vi "Authority Management.vi"() -> ()   [LabVIEW 2017]
uses:
  <vilib>/Utility/error.llb/DialogType.ctl
  Controls/Login Authority CSV FGV Command.ctl
  <vilib>/Utility/file.llb/Read From Spreadsheet File (string).vi
  Globle/Trigger Home Screen.vi
panel:
  in  "Cancel Button - Archive":bool
  in  "Delete":bool
  out "error out":errorcluster
  in  "error in (no error)":errorcluster
  in  "New":bool
  in  "Save":bool
  in  "Enable Disable":T1
  in  "SELECT AUTHORITY":string(combo)
  # "AUTHORITY ASSIGNMENT"
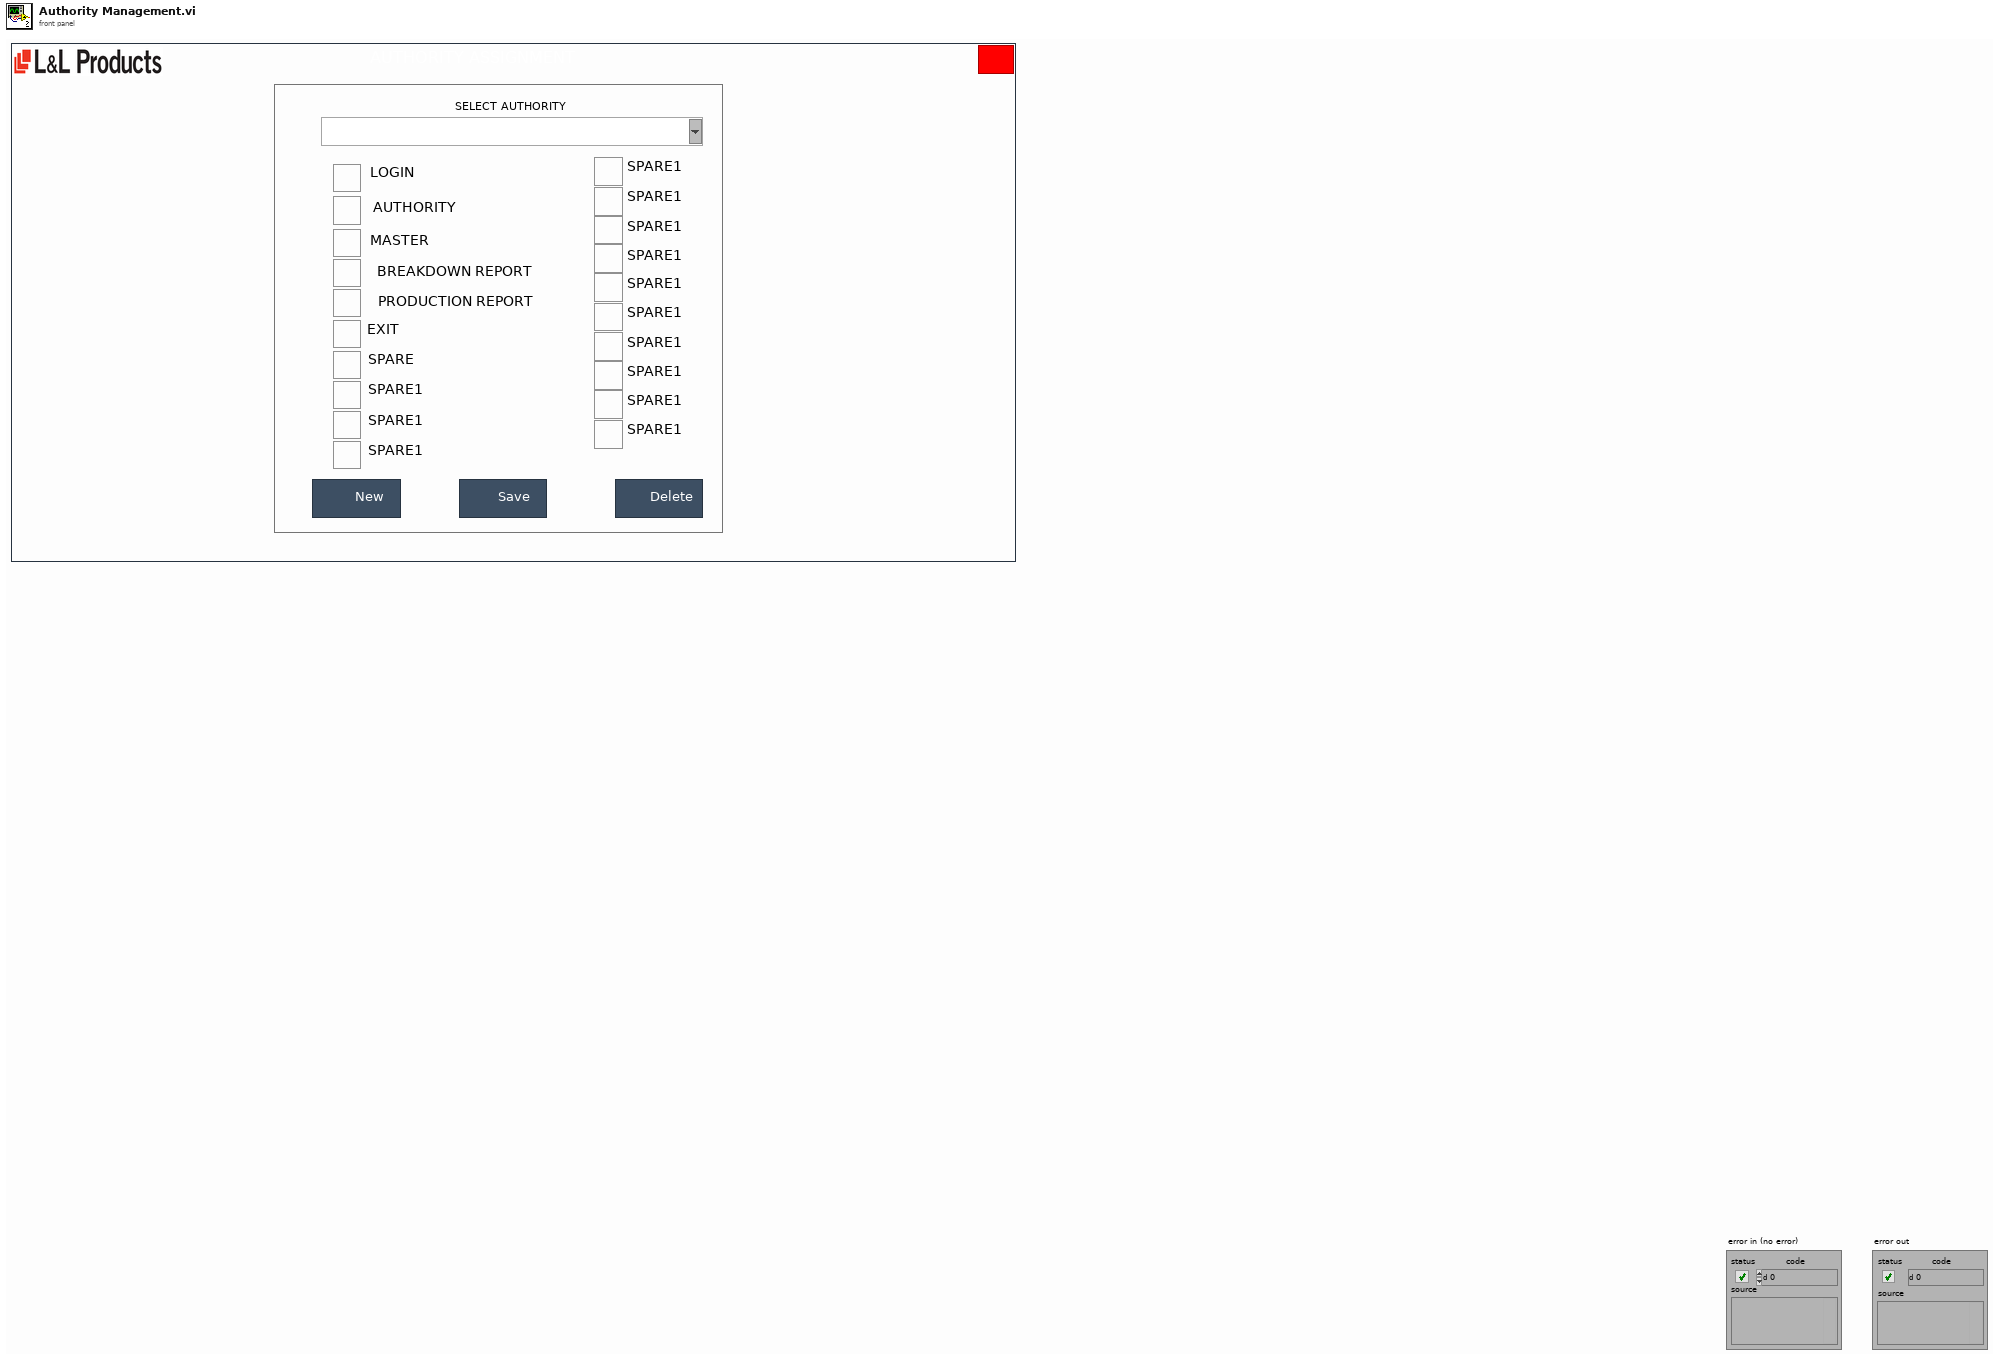
[diagram p1: front panel]
types:
  T1 = cluster{"SCREEN 1":bool, "SCREEN 2":bool, "SCREEN 3":bool, "SCREEN 4":bool, "SCREEN 5":bool, "SCREEN 6":bool, "SCREEN 7":bool, "SCREEN 8":bool, "SCREEN 9":bool, "SCREEN 10":bool, "SCREEN 11":bool, "SCREEN 12":bool, "SCREEN 13":bool, "SCREEN 14":bool, "SCREEN 15":bool, "SCREEN 16":bool, "SCREEN 17":bool, "SCREEN 18":bool, "SCREEN 19":bool, "SCREEN 20":bool}
  T2 = typedef "Login Authority CSV FGV Command.ctl" = enum16{"Init", "Save", "Read", "Get Data", "Delete"}
  T3 = typedef "DialogType.ctl" = u16
  T4 = enum32{"invalid app kind", "Development System", "Run Time System", "Student Edition", "Embedded LabVIEW", "Evaluation", "Custom"}
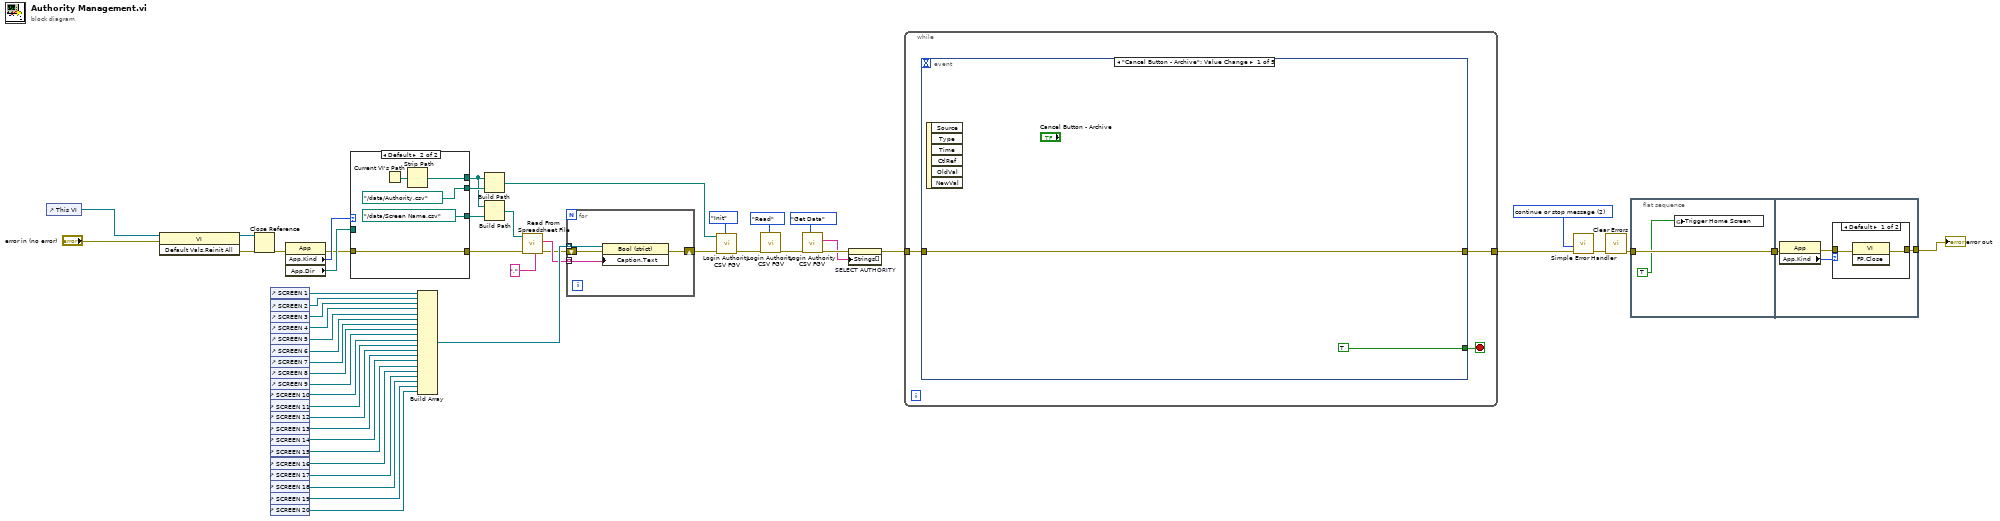
[diagram p0: block diagram]
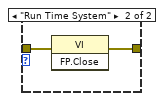
[diagram p2: hidden frame]
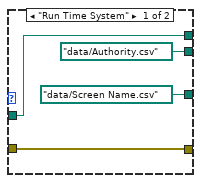
[diagram p3: hidden frame]
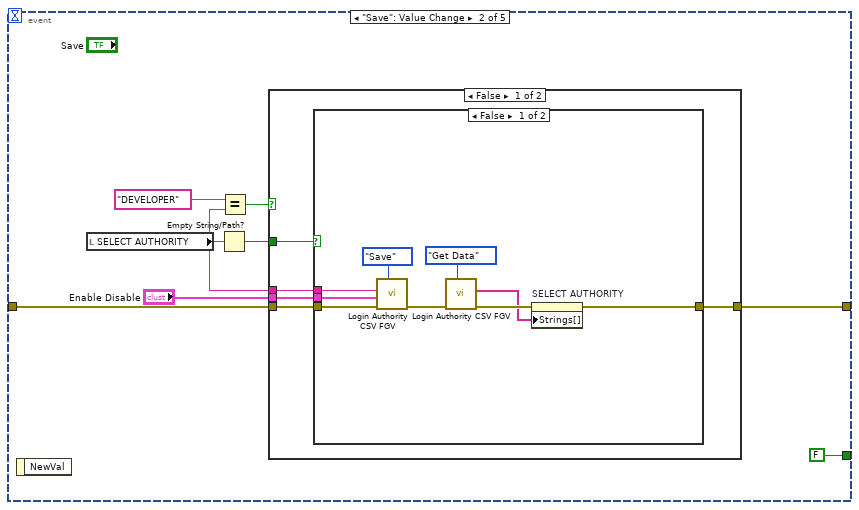
[diagram p4: hidden frame]
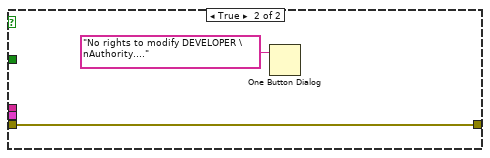
[diagram p6: hidden frame]
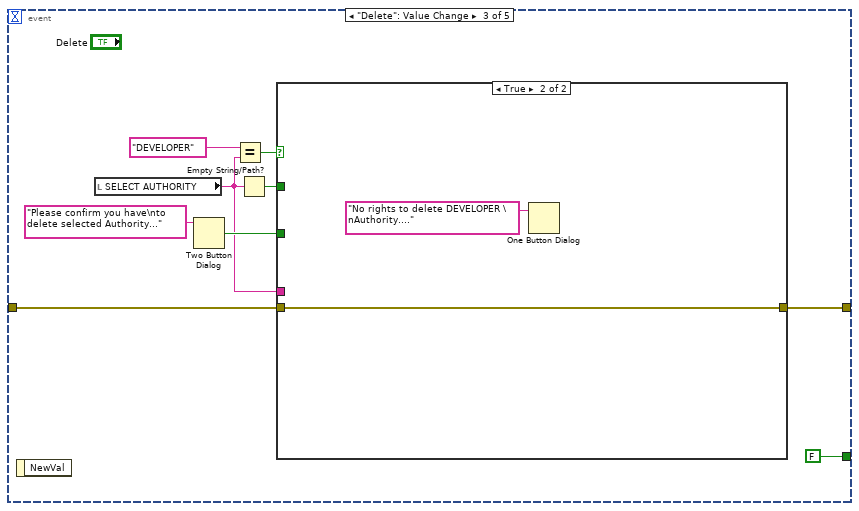
[diagram p7: hidden frame]
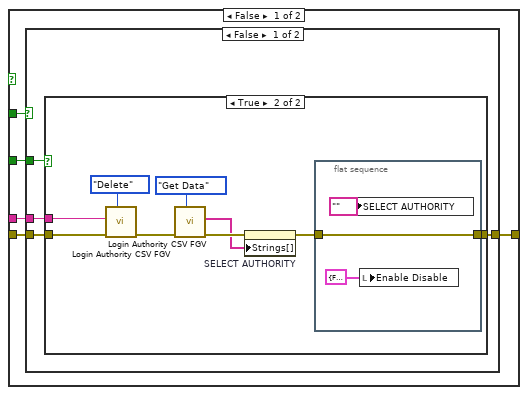
[diagram p8: hidden frame]
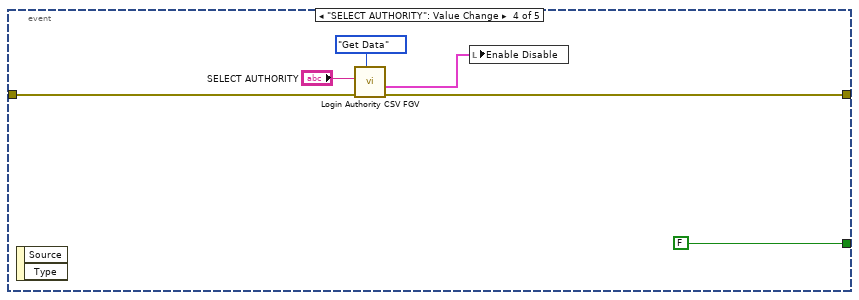
[diagram p11: hidden frame]
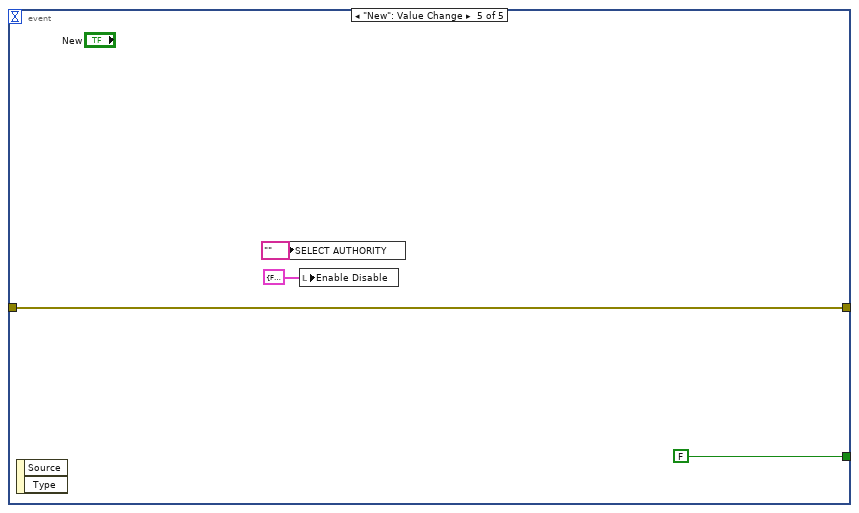
[diagram p12: hidden frame]
diagram:
  w41 = T3 2 items=["no dialog", "OK message", "continue or stop message", "OK message + warnings", "continue/stop + warnings"] ("type of dialog (OK msg:1)")
  n1 = control-ref of="This VI"() -> (w52:refnum<vi>)
  n2 = invoke class="VI" method="Default Vals.Reinit All"(reference=w52, error in="error in (no error)") -> (reference out=w49:refnum<vi>, error out=w50:errorcluster)  [unwired: 1 in, 1 out]
  n3 = Close Reference(reference=w49, error in (no error)=w50) -> (error out=w46:errorcluster)
  n4 = control-ref of="SCREEN 1"() -> (w27:refnum<vi>)
  n5 = control-ref of="SCREEN 2"() -> (w26:refnum<vi>)
  n6 = control-ref of="SCREEN 3"() -> (w25:refnum<vi>)
  n7 = control-ref of="SCREEN 4"() -> (w24:refnum<vi>)
  n8 = control-ref of="SCREEN 5"() -> (w23:refnum<vi>)
  n9 = control-ref of="SCREEN 6"() -> (w22:refnum<vi>)
  n10 = control-ref of="SCREEN 7"() -> (w21:refnum<vi>)
  n11 = control-ref of="SCREEN 8"() -> (w20:refnum<vi>)
  n12 = control-ref of="SCREEN 9"() -> (w19:refnum<vi>)
  n13 = control-ref of="SCREEN 10"() -> (w18:refnum<vi>)
  n14 = control-ref of="SCREEN 11"() -> (w17:refnum<vi>)
  n15 = control-ref of="SCREEN 12"() -> (w16:refnum<vi>)
  n16 = control-ref of="SCREEN 13"() -> (w15:refnum<vi>)
  n17 = control-ref of="SCREEN 14"() -> (w14:refnum<vi>)
  n18 = control-ref of="SCREEN 15"() -> (w13:refnum<vi>)
  n19 = control-ref of="SCREEN 16"() -> (w12:refnum<vi>)
  n20 = control-ref of="SCREEN 17"() -> (w11:refnum<vi>)
  n21 = control-ref of="SCREEN 18"() -> (w10:refnum<vi>)
  n22 = control-ref of="SCREEN 19"() -> (w5:refnum<vi>)
  n23 = control-ref of="SCREEN 20"() -> (w4:refnum<vi>)
  n24 = property class="App"(error in=w46) -> (error out=w45:errorcluster, "App.Kind"=w48:T4, "App.Dir"=w47:path)  [unwired: 1 in, 1 out]
  n25 = case shown="Default" w48 {
    tunnel: w47 -> [w56 _]
    tunnel: [path "data/Authority.csv" ("path") path "../data/Authority.csv" ("path")] -> w39
    tunnel: [w56 w59] -> w29
    tunnel: w45 -> [w54 w58]
    tunnel: [w54 w58] -> w2
    tunnel: [path "data/Screen Name.csv" ("path") path "../data/Screen Name.csv" ("path")] -> w28
    frame "Run Time System" {
    }
    frame Default {
      n26 = Current VI's Path() -> (path=w60:path)
      n27 = Strip Path(path=w60) -> (stripped path=w59:path)  [unwired: 1 out]
    }
  }
  n28 = Build Array(w27, w26, w25, w24, w23, w22, w21, w20, w19, w18, w17, w16, w15, w14, w13, w12, w11, w10, w5, w4) -> (w6:refnum<vi>[])
  n29 = Build Path(base path=w29, name or relative path=w39) -> (appended path=w38:path)
  n30 = Build Path(base path=w29, name or relative path=w28) -> (appended path=w9:path)
  n31 = call-poly <vilib>:"Read From Spreadsheet File.vi"("delimiter (\\t)"="," ("delimiter (\\t)"), "file path (dialog if empty)"=w9) -> ("first row"=w3:string[])  [unwired: 5 in, 4 out]
  n32 = for {
    shift-right: [w64] -> w7
    shift-left: w2 -> [w65]
    tunnel: w6 -> [w63] mode=indexing
    tunnel: w3 -> [w62] mode=indexing
    n33 = property class="Bool (strict)"(reference=w63, error in=w65, "Caption.Text"=w62) -> (error out=w64:errorcluster)  [unwired: 1 out]
  }
  n34 = call "Login Authority CSV FGV.vi"("Command"=Login_Authority_CSV_FGV_Command."Init", "error in (no error)"=w7, "Path"=w38) -> ("error out"=w34:errorcluster)  [unwired: 6 in, 2 out]
  n35 = call "Login Authority CSV FGV.vi"("Command"=Login_Authority_CSV_FGV_Command."Read", "error in (no error)"=w34) -> ("error out"=w33:errorcluster)  [unwired: 7 in, 2 out]
  n36 = call "Login Authority CSV FGV.vi"("Command"=Login_Authority_CSV_FGV_Command."Get Data", "error in (no error)"=w33) -> ("error out"=w32:errorcluster, "Authorities"=w30:string[])  [unwired: 7 in, 1 out]
  n37 = property on="SELECT AUTHORITY" class="CmbBox"(error in=w32, "Strings[]"=w30) -> (error out=w31:errorcluster)  [unwired: 1 in, 1 out]
  n38 = while {
    tunnel: w31 -> [w68]
    tunnel: [w67] -> w40
    stop <- w66 stop-if-true
    n39 = event shown="[0] \"Cancel Button - Archive\": Value Change" {
      selector: _ -> [_ _ _ _ _]
      dyn-events: _ -> [_ _ _ _ _]
      timeout: _ -> [_ _ _ _ _]
      tunnel: w68 -> [w70 w77 w103 w134 w137]
      tunnel: [w70 w75 w101 w133 w137] -> w67
      tunnel: [TRUE FALSE FALSE FALSE FALSE] -> w66
      event "Cancel Button - Archive": Value Change {
        n40 = event-data() -> ()  [unwired: 1 in, 6 out]
      }
      event "Save": Value Change {
        n41 = event-data() -> ()  [unwired: 1 in, 1 out]
        n42 = local read "SELECT AUTHORITY"() -> (w72:string)
        n43 = Empty String/Path?(string/path=w72) -> (empty?=w76:bool)
        n44 = Equal?(x="DEVELOPER", y=w72) -> (x = y?=w71:bool)
        n45 = case shown="False" w71 {
          tunnel: w77 -> [w83 w95]
          tunnel: w76 -> [w82 _]
          tunnel: [w81 w95] -> w75
          tunnel: w72 -> [w80 _]
          tunnel: "Enable Disable" -> [w79 _]
          frame False {
            n46 = case shown="False" w82 {
              tunnel: w83 -> [w91 w93]
              tunnel: [w85 w93] -> w81
              tunnel: w80 -> [w90 _]
              tunnel: w79 -> [w89 _]
              frame False {
                n47 = call "Login Authority CSV FGV.vi"("Command"=Login_Authority_CSV_FGV_Command."Save", "error in (no error)"=w91, "Data In"=w89, "Authority"=w90) -> ("error out"=w88:errorcluster)  [unwired: 5 in, 2 out]
                n48 = call "Login Authority CSV FGV.vi"("Command"=Login_Authority_CSV_FGV_Command."Get Data", "error in (no error)"=w88) -> ("error out"=w86:errorcluster, "Authorities"=w84:string[])  [unwired: 7 in, 1 out]
                n49 = property on="SELECT AUTHORITY" class="CmbBox"(error in=w86, "Strings[]"=w84) -> (error out=w85:errorcluster)  [unwired: 1 in, 1 out]
              }
              frame True {
              }
            }
          }
          frame True {
            n50 = One Button Dialog(message="No rights to modify DEVELOPER \nAuthority....") -> ()  [unwired: 1 in, 1 out]
          }
        }
      }
      event "Delete": Value Change {
        n51 = event-data() -> ()  [unwired: 1 in, 1 out]
        n52 = local read "SELECT AUTHORITY"() -> (w98:string)
        n53 = Two Button Dialog(message="Please confirm you have\nto delete selected Authority...") -> (T button?=w99:bool)  [unwired: 2 in]
        n54 = Equal?(x="DEVELOPER", y=w98) -> (x = y?=w96:bool)
        n55 = Empty String/Path?(string/path=w98) -> (empty?=w102:bool)
        n56 = case shown="True" w96 {
          tunnel: w103 -> [w109 w129]
          tunnel: w102 -> [w108 _]
          tunnel: [w107 w129] -> w101
          tunnel: w99 -> [w106 _]
          tunnel: w98 -> [w105 _]
          frame False {
            n57 = case shown="False" w108 {
              tunnel: w109 -> [w113 w127]
              tunnel: [w111 w127] -> w107
              tunnel: w105 -> [w112 _]
              tunnel: w106 -> [w110 _]
              frame False {
                n58 = case shown="True" w110 {
                  tunnel: w113 -> [w114 w122]
                  tunnel: w112 -> [_ w121]
                  tunnel: [w114 w115] -> w111
                  frame False {
                  }
                  frame True {
                    n59 = call "Login Authority CSV FGV.vi"("Command"=Login_Authority_CSV_FGV_Command."Delete", "error in (no error)"=w122, "Authority"=w121) -> ("error out"=w120:errorcluster)  [unwired: 6 in, 2 out]
                    n60 = call "Login Authority CSV FGV.vi"("Command"=Login_Authority_CSV_FGV_Command."Get Data", "error in (no error)"=w120) -> ("error out"=w118:errorcluster, "Authorities"=w117:string[])  [unwired: 7 in, 1 out]
                    n61 = property on="SELECT AUTHORITY" class="CmbBox"(error in=w118, "Strings[]"=w117) -> (error out=w116:errorcluster)  [unwired: 1 in, 1 out]
                    n62 = flat-sequence {
                      tunnel: w116 -> [w126]
                      tunnel: [w126] -> w115
                      frame #0 {
                        n63 = local write "SELECT AUTHORITY"("" ("AUTHORITY")) -> ()
                        n64 = local write "Enable Disable"(T1 {"SCREEN 1"=FALSE, "SCREEN 2"=FALSE, "SCREEN 3"=FALSE, "SCREEN 4"=FALSE, "SCREEN 5"=FALSE, "SCREEN 6"=FALSE, "SCREEN 7"=FALSE, "SCREEN 8"=FALSE, "SCREEN 9"=FALSE, "SCREEN 10"=FALSE, "SCREEN 11"=FALSE, "SCREEN 12"=FALSE, "SCREEN 13"=FALSE, "SCREEN 14"=FALSE, "SCREEN 15"=FALSE, "SCREEN 16"=FALSE, "SCREEN 17"=FALSE, "SCREEN 18"=FALSE, "SCREEN 19"=FALSE, "SCREEN 20"=FALSE} ("Enable Disable")) -> ()
                      }
                    }
                  }
                }
              }
              frame True {
              }
            }
          }
          frame True {
            n65 = One Button Dialog(message="No rights to delete DEVELOPER \nAuthority....") -> ()  [unwired: 1 in, 1 out]
          }
        }
      }
      event "SELECT AUTHORITY": Value Change {
        n66 = event-data() -> ()  [unwired: 1 in, 2 out]
        n67 = call "Login Authority CSV FGV.vi"("Command"=Login_Authority_CSV_FGV_Command."Get Data", "error in (no error)"=w134, "Authority"="SELECT AUTHORITY") -> ("error out"=w133:errorcluster, "Data Out"=w130:T1)  [unwired: 6 in, 1 out]
        n68 = local write "Enable Disable"(w130) -> ()
      }
      event "New": Value Change {
        n69 = event-data() -> ()  [unwired: 1 in, 2 out]
        n70 = local write "SELECT AUTHORITY"("" ("AUTHORITY")) -> ()
        n71 = local write "Enable Disable"(T1 {"SCREEN 1"=FALSE, "SCREEN 2"=FALSE, "SCREEN 3"=FALSE, "SCREEN 4"=FALSE, "SCREEN 5"=FALSE, "SCREEN 6"=FALSE, "SCREEN 7"=FALSE, "SCREEN 8"=FALSE, "SCREEN 9"=FALSE, "SCREEN 10"=FALSE, "SCREEN 11"=FALSE, "SCREEN 12"=FALSE, "SCREEN 13"=FALSE, "SCREEN 14"=FALSE, "SCREEN 15"=FALSE, "SCREEN 16"=FALSE, "SCREEN 17"=FALSE, "SCREEN 18"=FALSE, "SCREEN 19"=FALSE, "SCREEN 20"=FALSE} ("Enable Disable")) -> ()
      }
    }
  }
  n72 = call <vilib>:"Simple Error Handler.vi"("type of dialog (OK msg:1)"=w41, "error in (no error)"=w40) -> ("error out"=w44:errorcluster)  [unwired: 3 in, 4 out]
  n73 = call <vilib>:"Clear Errors.vi"("error in (no error)"=w44) -> ("error out"=w43:errorcluster)  [unwired: 5 in, 1 out]
  n74 = flat-sequence {
    tunnel: w43 -> [w141]
    tunnel: [w141] -> w1
    tunnel: [w142] -> w42
    tunnel: w1 -> [w143]
    frame #0 {
      n75 = global write "Trigger Home Screen.vi" "Trigger Home Screen"(TRUE ("Remove VI Edit User Subpanel")) -> ()
    }
    frame #1 {
      n76 = property class="App"(error in=w143) -> (error out=w144:errorcluster, "App.Kind"=w145:T4)  [unwired: 1 in, 1 out]
      n77 = case shown="Default" w145 {
        tunnel: w144 -> [w147 w149]
        tunnel: [w146 w148] -> w142
        frame Default {
          n78 = invoke class="VI" method="FP.Close"(error in=w147) -> (error out=w146:errorcluster)  [unwired: 2 in, 2 out]
        }
        frame "Run Time System" {
          n79 = invoke class="VI" method="FP.Close"(error in=w149) -> (error out=w148:errorcluster)  [unwired: 2 in, 2 out]
        }
      }
    }
  }
  "error out" <- w42
